vi "From I64.vi"   [LabVIEW 2017]
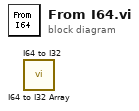
[diagram p0: block diagram]
diagram:
  n1 = call <vilib>:"I64 to I32 Array.vi"() -> ()  [unwired: 2 in, 2 out]
  n2 = call <vilib>:"I64 to I32.vi"() -> ()  [unwired: 2 in, 2 out]
